vi "写入合格信号.vi"(2 "信号":bool, 3 "设备号":string, 4 "产品ID":string) -> ()   [LabVIEW 2013]
uses:
  <vilib>/Utility/error.llb/whitespace.ctl
panel:
  in  "error in (no error)":errorcluster
  out "error out":errorcluster
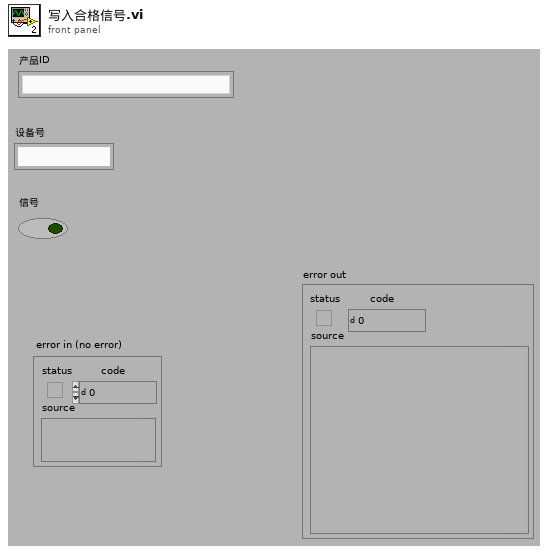
[diagram p1: front panel]
types:
  T1 = typedef "whitespace.ctl" = u16
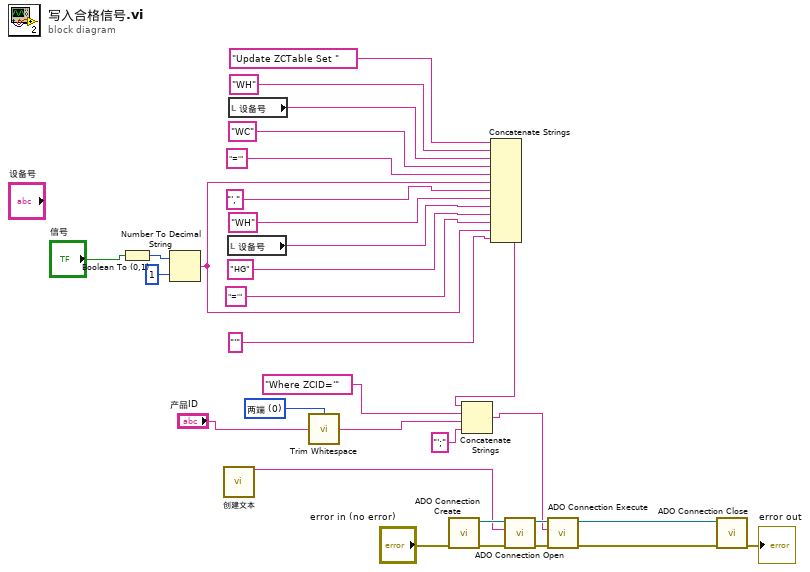
[diagram p0: block diagram]
diagram:
  w23 = T1 0 items=["两端", "字符串首端", "字符串末端"] ("location (both)")
  n1 = Boolean To (0,1)(Boolean="信号") -> (0, 1=w16:i16)
  n2 = Number To Decimal String(number=w16, width (-)=i16 1 ("宽度(-)")) -> (decimal integer string=w3:string)
  n3 = call "创建文本"() -> ("Result"=w19:string)  [unwired: 14 in, 1 out]
  n4 = local read "设备号"() -> (w6:string)
  n5 = local read "设备号"() -> (w11:string)
  n6 = call <vilib>:"Trim Whitespace.vi"("string"="产品ID", "location (both)"=w23) -> ("trimmed string"=w21:string)
  n7 = call "ADO Connection Create.vi"("error in (no error)"="error in (no error)") -> ("error out"=w30:errorcluster, "ADODB._Connection Out"=w31:refnum<k7>)  [unwired: 9 out]
  n8 = Concatenate Strings("Update ZCTable Set " ("字符串"), "WH", w11, "WC", "='", w3, "'," ("字符串"), "WH", w6, "HG", "='", w3, "'" ("字符串")) -> (w1:string)
  n9 = Concatenate Strings(w1, "Where ZCID='" ("字符串"), w21, "';" ("字符串")) -> (w18:string)
  n10 = call "ADO Connection Open.vi"("error in (no error)"=w30, "ConnectionString"=w19, "ADODB._Connection In"=w31) -> ("error out"=w29:errorcluster, "ADODB._Connection Out"=w28:refnum<k7>)  [unwired: 7 out]
  n11 = call "ADO Connection Execute.vi"("error in (no error)"=w29, "CommandText"=w18, "ADODB._Connection In"=w28) -> ("error out"=w24:errorcluster, "ADODB._Connection Out"=w27:refnum<k7>)  [unwired: 7 out]
  n12 = call "ADO Connection Close.vi"("error in (no error)"=w24, "ADODB._Connection In"=w27) -> ("error out"=→"error out":errorcluster)  [unwired: 9 out]
